vi "Global 1.vi"() -> ()   [LabVIEW 2017]
panel:
  in  "Stop Button":bool
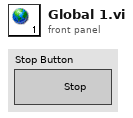
[diagram p1: front panel]
diagram:
